vi "New.vi"(5 "Extension":string="mustache", 6 "Search Path":path[](array[path]), 7 "Root":path=path "", 8 "Error In":errorcluster) -> (0 "Error Out":errorcluster, 3 "File":refnum<class "File.lvclass">)   [LabVIEW 2018, in "Toolkit.lvlib" / "Loaders.lvlib" / "File.lvclass"]
doc: "Creates a new <B>File</B> partial loader object. The key for a partial tag is a file name without the extension.\n\n<B>Root</B> - The folder containing all Mustache templates. If <Not A Path> or empty, then partial Mustache templates will be searched using the Search Path.\n\n<B>Search Path</B> - An array of folders to search for partial Mustache templates. The key for a partial tag is the file name.\n\n<B>Extension</B> - The file extension for partial Mustache templates stored in files on disk.\n\n<B>File</B> - Represents a partial loader of Mustache templates that uses the key to a partial tag as a file a name loads the Mustache template from the matching file."
uses:
  File.lvclass
  File.lvclass/File.ctl
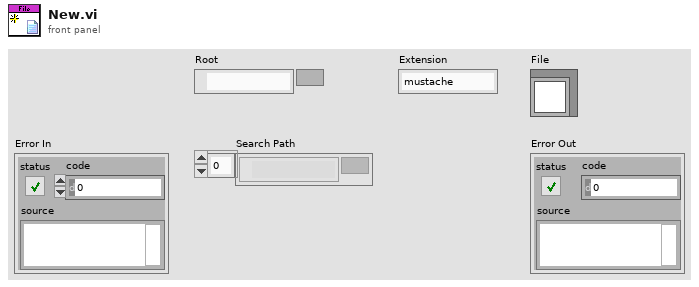
[diagram p1: front panel]
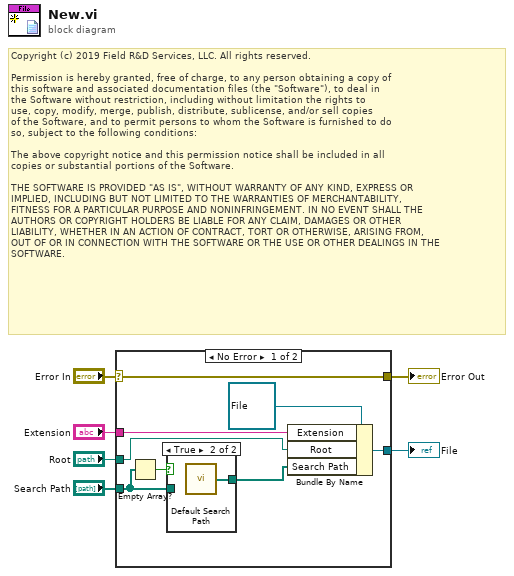
[diagram p0: block diagram]
diagram:
  # "Copyright (c) 2019 Field R&D Services, LLC. All rights reserved.\n\nPermission is hereby granted, free of charge, to any person obtaining a copy of\nthis software and associated documentation files (the \"Software\"), to deal in\nthe Software without restriction, including without limitation the rights to\nuse, copy, modify, merge, publish, distribute, sublicense, and/or sell copies\nof the Software, and to permit persons to whom the Software is furnished to do\nso, subject to the following conditions:\n\nThe above copyright notice and this permission notice shall be included in all\ncopies or substantial portions of the Software.\n\nTHE SOFTWARE IS PROVIDED \"AS IS\", WITHOUT WARRANTY OF ANY KIND, EXPRESS OR\nIMPLIED, INCLUDING BUT NOT LIMITED TO THE WARRANTIES OF MERCHANTABILITY,\nFITNESS FOR A PARTICULAR PURPOSE AND NONINFRINGEMENT. IN NO EVENT SHALL THE\nAUTHORS OR COPYRIGHT HOLDERS BE LIABLE FOR ANY CLAIM, DAMAGES OR OTHER\nLIABILITY, WHETHER IN AN ACTION OF CONTRACT, TORT OR OTHERWISE, ARISING FROM,\nOUT OF OR IN CONNECTION WITH THE SOFTWARE OR THE USE OR OTHER DEALINGS IN THE\nSOFTWARE."
  n1 = case shown="No Error" "Error In" {
    selector: "Error In" -> [w7 w17]
    tunnel: "Extension" -> [w13 _]
    tunnel: "Root" -> [w12 _]
    tunnel: [w10 _] -> w4
    tunnel: "Search Path" -> [w9 _]
    tunnel: [w7 w17] -> w1
    frame No Error {
      n2 = Empty Array?(array=w9) -> (empty?=w8:bool)
      n3 = case shown="True" w8 {
        tunnel: [w15 w16] -> w11
        tunnel: w9 -> [w15 _]
        frame False {
        }
        frame True {
          n4 = call "Default Search Path.vi"() -> ("Search Path"=w16:path[])
        }
      }
      n5 = Bundle By Name(cluster=refnum<class "File.lvclass"> refnum ("Toolkit.lvlib:Loaders.lvlib:File.lvclass"), "Extension"=w13, "Root"=w12, "Search Path"=w11) -> (w10:refnum<class "File.lvclass">)
    }
    frame Error {
    }
  }
  "File" <- w4
  "Error Out" <- w1
